vi "Versuchsaufbau anlegen.vi"(6 "error in (no error)":errorcluster, 9 "Data":T1={"Report.lvclass"=refnum, "test"="", "last State"=enum."Initialize", "test ID"=0, "parameter"=[], "EMTestCWS500N.lvclass"=refnum, "CEG4500.lvclass"=refnum, "Tektronix RSA5106A.lvclass"=refnum, "erfolgreich"=FALSE, "log"="", "Kommentar"="", "Device Enum"=enum."emTestCWS500N", "Test Enum"=enum."HF-Felder", "debug"=FALSE}) -> (0 "error out 2":errorcluster caption="error out", 2 "Setup Ausgang":refnum<class "Setup.lvclass">, 3 "Abbrechen out":bool)   [LabVIEW 2013, in "DataCreation.lvlib"]
uses:
  lib/DataCreation.lvlib
  Main/controls/Data.ctl
  classes/Datastructure/Report/Report.lvclass
  classes/Devices/emTestCWS500N/EMTestCWS500N.lvclass
  classes/Devices/CEG4500/CEG4500.lvclass
  classes/Devices/Tektronix RSA5106A/Tektronix RSA5106A.lvclass
  Main/controls/State.ctl
  classes/Devices/DeviceInterface/Devices.ctl
  classes/Tests/TestInterface/Tests.ctl
  classes/Datastructure/Setup/Setup.lvclass
  classes/Datastructure/Image/img.lvclass
  classes/Datastructure/Device/Device.lvclass
  lib/TreeRepresentation.lvlib
panel:
  in  "number of devices":i32
  in  "number of pictures":i32
  in  "Tab Control":enum32{"Versuchsaufbau", "Daten"}(tab)
  in  "Abbrechen":bool
  in  "Tree 2":string(tree)
  out "Titel":string caption="Test"
  in  "OK Button":bool
  in  "Add picture":bool
  in  "Kommentar":string
  in  "Add Device":bool
  in  "Tree":string(tree)
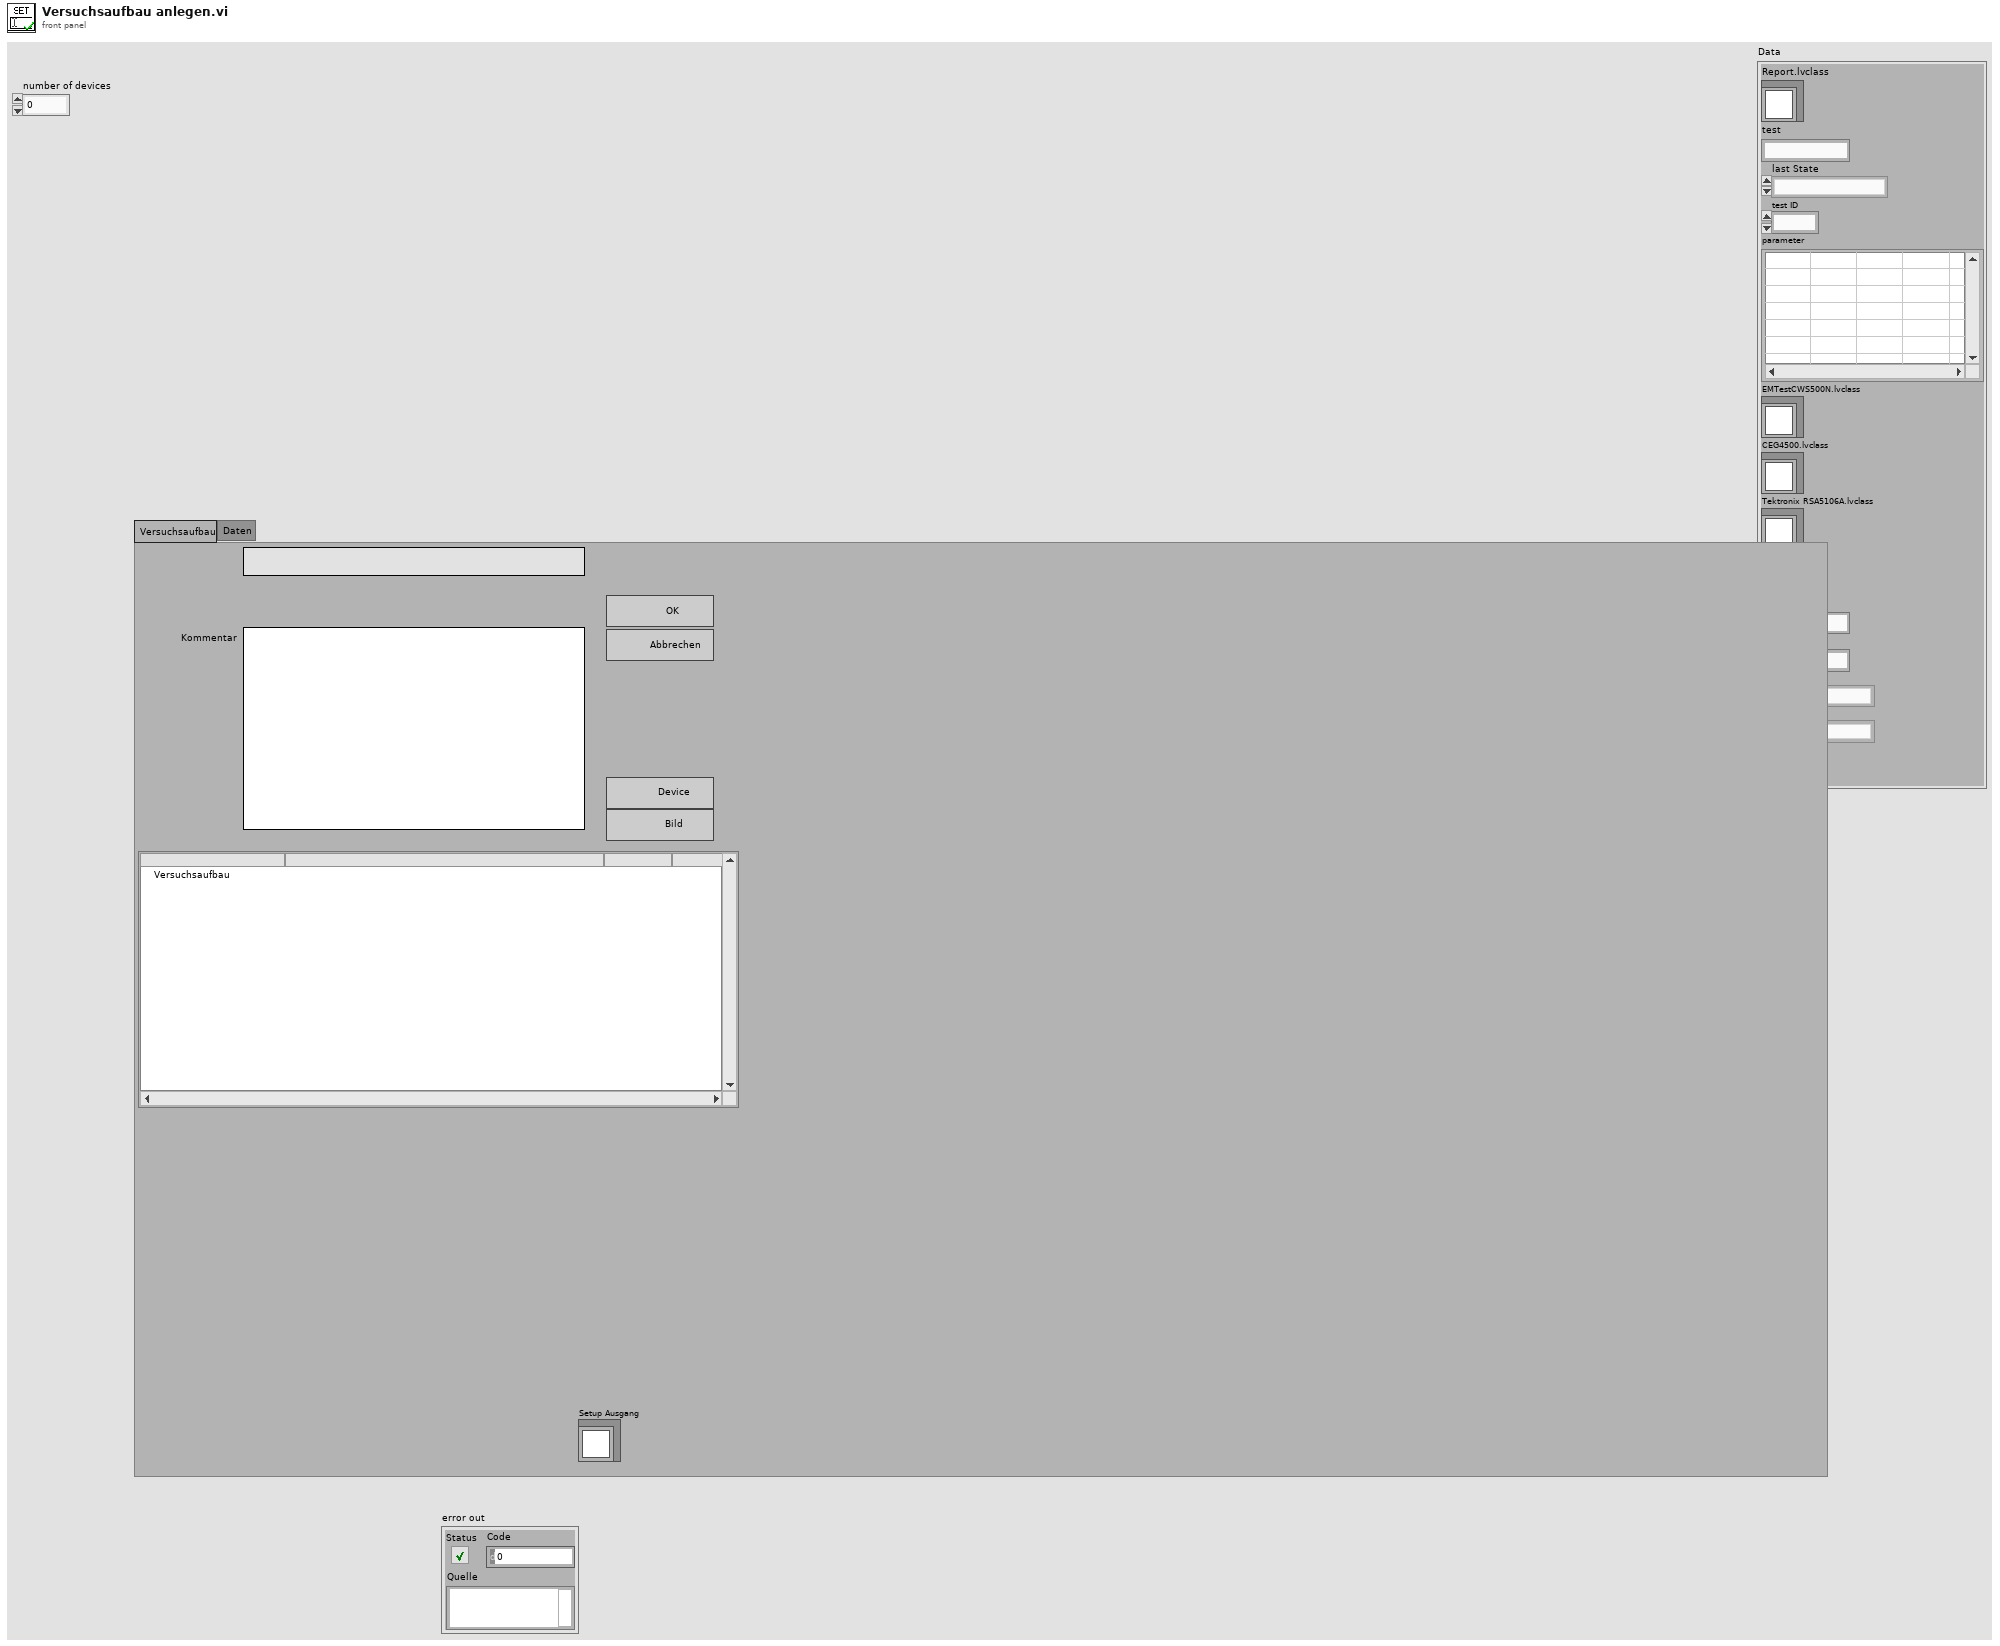
[diagram p1: front panel]
types:
  T1 = typedef "Data.ctl" = cluster{"Report.lvclass":refnum<class "Report.lvclass">, "test":string, "last State":T2, "test ID":i32, "parameter":string[][], "EMTestCWS500N.lvclass":refnum<class "EMTestCWS500N.lvclass">, "CEG4500.lvclass":refnum<class "CEG4500.lvclass">, "Tektronix RSA5106A.lvclass":refnum<class "Tektronix RSA5106A.lvclass">, "erfolgreich":bool, "log":string, "Kommentar":string, "Device Enum":T3, "Test Enum":T4, "debug":bool}
  T2 = typedef "State.ctl" = enum16{"create Pdf", "load Report", "save Report", "do Test", "CDN Kalibrierung", "enter Report Parameters", "new Test", "Protokoll", "read Tree", "update Tree", "Fehler", "Initialize", "Wait for Event", "Exit"}
  T3 = typedef "Devices.ctl" = enum16{"unbekannt", "Tektronix RSA5106A", "emTestCWS500N", "CEG-4500"}
  T4 = typedef "Tests.ctl" = enum16{"unbekannt", "Störaussendung", "Burst", "ESD", "Surge", "Spannungseinbruch", "HF-Felder"}
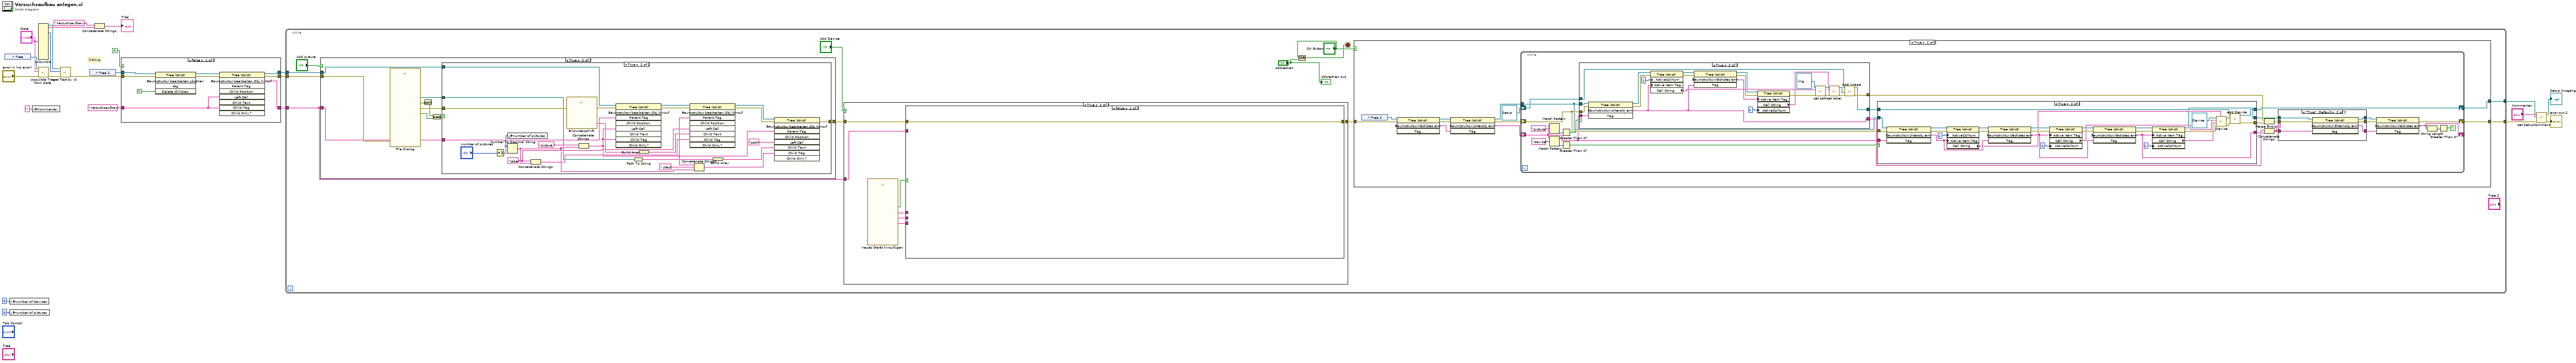
[diagram p0: block diagram]
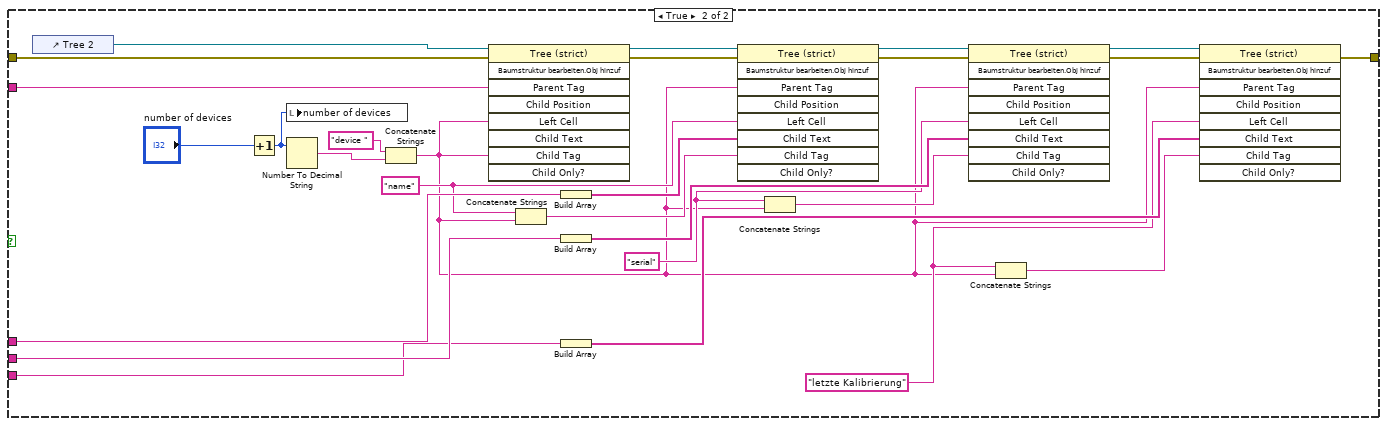
[diagram p4: hidden frame]
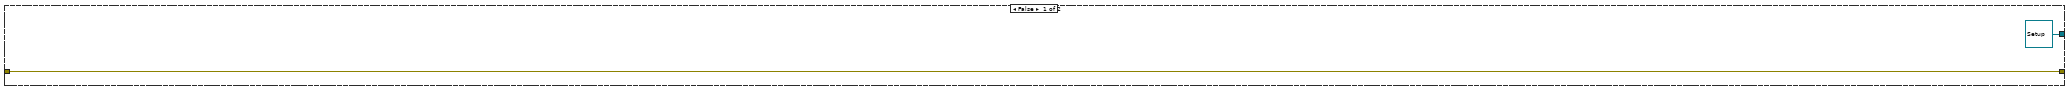
[diagram p5: hidden frame]
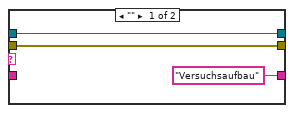
[diagram p6: hidden frame]
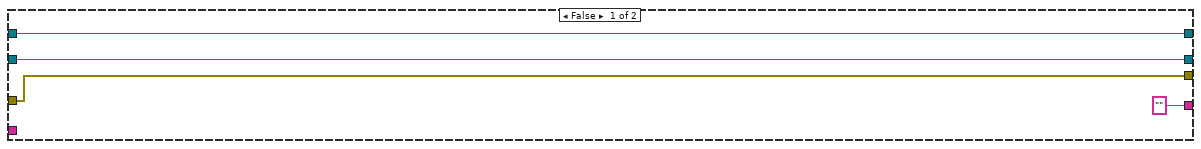
[diagram p7: hidden frame]
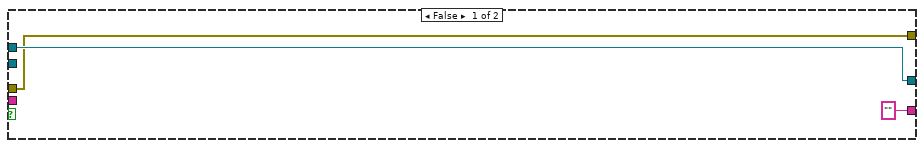
[diagram p8: hidden frame]
diagram:
  # "Debug"
  n1 = control-ref of="Tree"() -> (w24:refnum<vi>)
  n2 = local write "number of devices"(0 ("number of devices")) -> ()
  n3 = local write "number of pictures"(0 ("number of devices")) -> ()
  n4 = local write "Kommentar"("" ("Kommentar")) -> ()
  n5 = Unbundle("Data") -> ("Report.lvclass"=w19:refnum<class "Report.lvclass">, "test"=w20:string, "test ID"=w16:i32)  [unwired: 11 out]
  n6 = call "populate Tree from Data.vi"("error in (no error)"="error in (no error)", "Data"="Data", "reference"=w24) -> ("error out"=w18:errorcluster)  [unwired: 6 in]
  n7 = call-dynamic "get Test by id.vi"("error in (no error)"=w18, "id"=w16, "Report (Eingang)"=w19) -> ("error out"=w12:errorcluster)  [unwired: 4 in, 4 out]
  n8 = control-ref of="Tree 2"() -> (w11:refnum<vi>)
  n9 = Concatenate Strings("Versuchsaufbau ", w20) -> (→"Titel":string)
  n10 = case shown="False" FALSE {
    tunnel: "Versuchsaufbau" ("Elternobjekt-Tag") -> [w33 w34]
    tunnel: [w32 w34] -> w14
    tunnel: [w31 w36] -> w13
    tunnel: w12 -> [w30 w36]
    tunnel: w11 -> [w29 w35]
    tunnel: [w28 w35] -> w10
    frame False {
      n11 = invoke on="Invoke Node" class="Tree (strict)" method="Baumstruktur bearbeiten.Löschen"(reference=w29, error in=w30, "Delete Children"=TRUE ("Unterobjekte löschen?")) -> (reference out=w27:refnum<vi>, error out=w26:errorcluster)  [unwired: 2 in, 3 out]
      n12 = invoke class="Tree (strict)" method="Baumstruktur bearbeiten.Obj hinzuf"(reference=w27, error in=w26, "Left Cell"=w33, "Child Tag"=w33) -> (reference out=w28:refnum<vi>, error out=w31:errorcluster, "Edit Tree Items:Add Item"=w32:string)  [unwired: 5 in, 6 out]
    }
    frame True {
    }
  }
  n13 = while {
    tunnel: w13 -> [w44]
    tunnel: w14 -> [w43]
    tunnel: w10 -> [w42]
    tunnel: [w41] -> w5
    tunnel: [w40] -> w7
    stop <- w38 stop-if-true
    n14 = case shown="True" "Add picture" {
      tunnel: [w194 w202] -> w46
      tunnel: w44 -> [w194 w201]
      tunnel: w43 -> [_ w200]
      tunnel: w42 -> [_ w199]
      frame False {
      }
      frame True {
        n15 = call "File Dialog"("error in"=w201) -> ("selected path"=w204:path, "exists"=w195:bool, "cancelled"=w198:bool, "error out"=w203:errorcluster)  [unwired: 11 in]
        n16 = Not(x=w198) -> (.not. x?=w196:bool)
        n17 = And(x=w196, y=w195) -> (x .and. y?=w197:bool)
        n18 = case shown="True" w197 {
          tunnel: w204 -> [_ w221]
          tunnel: w203 -> [w205 w216]
          tunnel: [w205 w208] -> w202
          tunnel: w200 -> [_ w207]
          tunnel: w199 -> [_ w206]
          frame False {
          }
          frame True {
            w224 = "label" ("Left Cell String")
            n19 = Increment(x="number of pictures") -> (x+1=w212:i32)
            n20 = local write "number of pictures"(w212) -> ()
            n21 = Number To Decimal String(number=w212) -> (decimal integer string=w223:string)  [unwired: 1 in]
            n22 = Concatenate Strings(w224, w223) -> (w222:string)
            n23 = call "Bildunterschrift"("error in (no error)"=w216) -> ("Bildunterschrift"=w215:string, "error out"=w211:errorcluster)  [unwired: 16 in, 1 out]
            n24 = Concatenate Strings("picture " ("Left Cell String"), w223) -> (w225:string)
            n25 = invoke class="Tree (strict)" method="Baumstruktur bearbeiten.Obj hinzuf"(reference=w206, error in=w211, "Parent Tag"=w207, "Left Cell"=w225, "Child Tag"=w225) -> (reference out=w219:refnum<vi>, error out=w210:errorcluster)  [unwired: 4 in, 7 out]
            n26 = Path To String(path=w221) -> (string=w217:string)
            n27 = Build Array(w215) -> (w214:string[])
            n28 = invoke class="Tree (strict)" method="Baumstruktur bearbeiten.Obj hinzuf"(reference=w219, error in=w210, "Parent Tag"=w225, "Left Cell"=w224, "Child Text"=w214, "Child Tag"=w222) -> (reference out=w218:refnum<vi>, error out=w209:errorcluster)  [unwired: 3 in, 7 out]
            n29 = Concatenate Strings(w225, " pfad", w223) -> (w227:string)
            n30 = Build Array(w217) -> (w220:string[])
            n31 = invoke class="Tree (strict)" method="Baumstruktur bearbeiten.Obj hinzuf"(reference=w218, error in=w209, "Parent Tag"=w225, "Left Cell"="path" ("Left Cell String"), "Child Text"=w220, "Child Tag"=w227) -> (error out=w208:errorcluster)  [unwired: 3 in, 8 out]
          }
        }
      }
    }
    n32 = case shown="True" "Add Device" {
      tunnel: [w49 w51] -> w45
      tunnel: w46 -> [w49 w55]
      tunnel: w43 -> [_ w56]
      frame False {
      }
      frame True {
        n33 = call "neues Gerät hinzufügen"() -> ("letzte Kalibrierung"=w52:string, "Seriennummer"=w53:string, "Device name"=w54:string, "OK"=w50:bool)  [unwired: 15 in, 1 out]
        n34 = case shown="False" w50 {
          tunnel: w56 -> [_ w79]
          tunnel: w55 -> [w57 w78]
          tunnel: w54 -> [_ w71]
          tunnel: w53 -> [_ w70]
          tunnel: w52 -> [_ w69]
          tunnel: [w57 w58] -> w51
          frame False {
          }
          frame True {
            w61 = "letzte Kalibrierung" ("Linker Zellen-String")
            w63 = "serial" ("Linker Zellen-String")
            w65 = "name" ("Linker Zellen-String")
            n35 = control-ref of="Tree 2"() -> (w84:refnum<vi>)
            n36 = Increment(x="number of devices") -> (x+1=w80:i32)
            n37 = local write "number of devices"(w80) -> ()
            n38 = Number To Decimal String(number=w80) -> (decimal integer string=w82:string)  [unwired: 1 in]
            n39 = Concatenate Strings("device " ("Left Cell String"), w82) -> (w60:string)
            n40 = invoke class="Tree (strict)" method="Baumstruktur bearbeiten.Obj hinzuf"(reference=w84, error in=w78, "Parent Tag"=w79, "Left Cell"=w60, "Child Tag"=w60) -> (reference out=w76:refnum<vi>, error out=w77:errorcluster)  [unwired: 4 in, 7 out]
            n41 = Concatenate Strings(w65, w60) -> (w64:string)
            n42 = Build Array(w71) -> (w68:string[])
            n43 = Build Array(w70) -> (w67:string[])
            n44 = Build Array(w69) -> (w66:string[])
            n45 = invoke class="Tree (strict)" method="Baumstruktur bearbeiten.Obj hinzuf"(reference=w76, error in=w77, "Parent Tag"=w60, "Left Cell"=w65, "Child Text"=w68, "Child Tag"=w64) -> (reference out=w75:refnum<vi>, error out=w74:errorcluster)  [unwired: 3 in, 7 out]
            n46 = Concatenate Strings(w63, w60) -> (w62:string)
            n47 = invoke class="Tree (strict)" method="Baumstruktur bearbeiten.Obj hinzuf"(reference=w75, error in=w74, "Parent Tag"=w60, "Left Cell"=w63, "Child Text"=w67, "Child Tag"=w62) -> (reference out=w72:refnum<vi>, error out=w73:errorcluster)  [unwired: 3 in, 7 out]
            n48 = Concatenate Strings(w61, w60) -> (w59:string)
            n49 = invoke class="Tree (strict)" method="Baumstruktur bearbeiten.Obj hinzuf"(reference=w72, error in=w73, "Parent Tag"=w60, "Left Cell"=w61, "Child Text"=w66, "Child Tag"=w59) -> (error out=w58:errorcluster)  [unwired: 3 in, 8 out]
          }
        }
      }
    }
    n50 = Or(x="OK Button", y="Abbrechen") -> (x .or. y?=w38:bool)
    n51 = case shown="True" "OK Button" {
      tunnel: [refnum<class "Setup.lvclass"> refnum ("Setup Ausgang") w96] -> w40
      tunnel: [w86 w97] -> w41
      tunnel: w45 -> [w86 w94]
      frame False {
      }
      frame True {
        n52 = control-ref of="Tree 2"() -> (w93:refnum<vi>)
        n53 = invoke class="Tree (strict)" method="Baumstruktur.Nächstes erm"(reference=w93, error in=w94) -> (reference out=w92:refnum<vi>, error out=w91:errorcluster, "Navigate Tree:Get Next Item"=w90:string)  [unwired: 2 in, 1 out]
        n54 = invoke class="Tree (strict)" method="Baumstruktur.Unterobj erm"(reference=w92, error in=w91, "Tag"=w90) -> (reference out=w87:refnum<vi>, error out=w89:errorcluster, "Navigate Tree:Get Child"=w88:string)  [unwired: 1 in, 1 out]
        n55 = while {
          shift-right: [w101] -> w97
          shift-left: w89 -> [w117]
          shift-right: [w110] -> w96
          shift-left: refnum<class "Setup.lvclass"> refnum ("Setup Ausgang") -> [w116]
          shift-right: [w99] -> _
          shift-left: w88 -> [w114]
          tunnel: w87 -> [w115]
          stop <- w104 continue-if-true
          n56 = Match Pattern(string=w114, regular expression="picture" ("Regulärer Ausdruck")) -> (offset past match=w122:i32)  [unwired: 1 in, 3 out]
          n57 = Match Pattern(string=w114, regular expression="device" ("Regulärer Ausdruck")) -> (offset past match=w118:i32)  [unwired: 1 in, 3 out]
          n58 = Greater Than 0?(x=w122) -> (x > 0?=w121:bool)
          n59 = Greater Than 0?(x=w118) -> (x > 0?=w120:bool)
          n60 = case shown="True" w121 {
            tunnel: w114 -> [_ w172]
            tunnel: w117 -> [w167 w173]
            tunnel: w115 -> [_ w174]
            tunnel: [w167 w178] -> w109
            tunnel: w116 -> [w168 w177]
            tunnel: [w168 w171] -> w111
            tunnel: ["" ("Navigate Tree:Get Child") w170] -> w113
            frame False {
            }
            frame True {
              n61 = invoke class="Tree (strict)" method="Baumstruktur.Unterobj erm"(reference=w174, error in=w173, "Tag"=w172) -> (reference out=w176:refnum<vi>, error out=w175:errorcluster, "Navigate Tree:Get Child"=w170:string)  [unwired: 1 in, 1 out]
              n62 = property class="Tree (strict)"(reference=w176, error in=w175, "ActiveColNum"=1 ("Active Cell:Active Column Number"), "Active Item Tag"=w170) -> (reference out=w186:refnum<vi>, error out=w187:errorcluster, "Cell String"=w182:string)
              n63 = invoke class="Tree (strict)" method="Baumstruktur.Nächstes erm"(reference=w186, error in=w187, "Tag"=w170) -> (reference out=w185:refnum<vi>, error out=w184:errorcluster, "Navigate Tree:Get Next Item"=w181:string)  [unwired: 1 in, 1 out]
              n64 = property class="Tree (strict)"(reference=w185, error in=w184, "Active Item Tag"=w181, "ActiveColNum"=1 ("Active Cell:Active Column Number")) -> (error out=w191:errorcluster, "Cell String"=w183:string)  [unwired: 1 out]
              n65 = call-dynamic "set path.vi"("error in (no error)"=w191, "path"=w182, "img (Eingang)"=refnum<class "img.lvclass"> refnum ("img.lvclass")) -> ("error out"=w190:errorcluster, "img (Ausgang)"=w188:refnum<class "img.lvclass">)  [unwired: 7 in]
              n66 = call-dynamic "set label.vi"("error in (no error)"=w190, "label"=w183, "img (Eingang)"=w188) -> ("error out"=w192:errorcluster, "img (Ausgang)"=w193:refnum<class "img.lvclass">)  [unwired: 7 in]
              n67 = call-dynamic "add image.vi"("error in (no error)"=w192, "img.lvclass"=w193, "Setup (Eingang)"=w177) -> ("error out"=w178:errorcluster, "Setup (Ausgang)"=w171:refnum<class "Setup.lvclass">)  [unwired: 7 in]
            }
          }
          n68 = case shown="True" w120 {
            tunnel: w117 -> [w134 w159]
            tunnel: w115 -> [w133 w158]
            tunnel: w114 -> [_ w156]
            tunnel: ["" ("Navigate Tree:Get Next Item") w147] -> w112
            tunnel: w111 -> [w135 w141]
            tunnel: [w134 w142] -> w108
            tunnel: [w135 w140] -> w110
            tunnel: [w133 w139] -> w106
            frame False {
            }
            frame True {
              n69 = invoke class="Tree (strict)" method="Baumstruktur.Unterobj erm"(reference=w158, error in=w159, "Tag"=w156) -> (reference out=w157:refnum<vi>, error out=w160:errorcluster, "Navigate Tree:Get Child"=w155:string)  [unwired: 1 in, 1 out]
              n70 = property class="Tree (strict)"(reference=w157, error in=w160, "ActiveColNum"=1 ("Active Cell:Active Column Number"), "Active Item Tag"=w155) -> (reference out=w165:refnum<vi>, error out=w166:errorcluster, "Cell String"=w137:string)
              n71 = invoke class="Tree (strict)" method="Baumstruktur.Nächstes erm"(reference=w165, error in=w166, "Tag"=w155) -> (reference out=w164:refnum<vi>, error out=w163:errorcluster, "Navigate Tree:Get Next Item"=w148:string)  [unwired: 1 in, 1 out]
              n72 = property class="Tree (strict)"(reference=w164, error in=w163, "Active Item Tag"=w148, "ActiveColNum"=1 ("Active Cell:Active Column Number")) -> (reference out=w153:refnum<vi>, error out=w154:errorcluster, "Cell String"=w149:string)
              n73 = invoke class="Tree (strict)" method="Baumstruktur.Nächstes erm"(reference=w153, error in=w154, "Tag"=w148) -> (reference out=w152:refnum<vi>, error out=w151:errorcluster, "Navigate Tree:Get Next Item"=w147:string)  [unwired: 1 in, 1 out]
              n74 = property class="Tree (strict)"(reference=w152, error in=w151, "Active Item Tag"=w147, "ActiveColNum"=1 ("Aktive Zelle:Nummer der aktiven Spalte")) -> (reference out=w139:refnum<vi>, error out=w146:errorcluster, "Cell String"=w138:string)
              n75 = call-dynamic "Device.vi"("last calibration"=w137, "error in (no error)"=w146, "Name"=w138, "serial"=w149, "Device Eingang"=refnum<class "Device.lvclass"> refnum ("Device.lvclass")) -> ("error out"=w143:errorcluster, "Device Ausgang"=w144:refnum<class "Device.lvclass">)  [unwired: 5 in]
              n76 = call-dynamic "add Device.vi"("error in (no error)"=w143, "Device.lvclass"=w144, "Setup Eingang"=w141) -> ("error out"=w142:errorcluster, "Setup Ausgang"=w140:refnum<class "Setup.lvclass">)  [unwired: 7 in]
            }
          }
          n77 = Merge Errors(w109, w108) -> (w107:errorcluster)
          n78 = Concatenate Strings(w113, w112) -> (w98:string)
          n79 = case shown="\"True\", Default" w98 {
            tunnel: w107 -> [w126 w132]
            tunnel: w106 -> [w125 w131]
            tunnel: w98 -> [_ w130]
            tunnel: [w126 w129] -> w103
            tunnel: [w125 w128] -> w102
            tunnel: ["Versuchsaufbau" ("Navigate Tree:Get Parent") w127] -> w100
            frame "" {
            }
            frame "True", Default {
              n80 = invoke class="Tree (strict)" method="Baumstruktur.Elternobj erm"(reference=w131, error in=w132, "tag"=w130) -> (reference out=w128:refnum<vi>, error out=w129:errorcluster, "Navigate Tree:Get Parent"=w127:string)  [unwired: 1 in, 1 out]
            }
          }
          n81 = invoke class="Tree (strict)" method="Baumstruktur.Nächstes erm"(reference=w102, error in=w103, "Tag"=w100) -> (error out=w101:errorcluster, "Navigate Tree:Get Next Item"=w99:string)  [unwired: 1 in, 2 out]
          n82 = String Length(string=w99) -> (length=w105:i32)
          n83 = Greater Than 0?(x=w105) -> (x > 0?=w104:bool)
        }
      }
    }
    "Abbrechen out" <- "Abbrechen"
  }
  n84 = call-dynamic "set SetupComment.vi"("error in (no error)"=w5, "Comment"="Kommentar", "Setup (Eingang)"=w7) -> ("error out"=→"error out 2":errorcluster, "Setup (Ausgang)"=→"Setup Ausgang":refnum<class "Setup.lvclass">)  [unwired: 7 in]
